vi "Read Heater and Valve.vi"(8 "error in (no error)":errorcluster, 11 "Temperature Controller in":refnum<class "Temperature Controller.lvclass">) -> (0 "error out":errorcluster, 1 "valve%":T2 caption="Valve" max=100.0 scale=0.0..100.0 scale format="%.1f", 2 "heater%":T2 caption="Heater" max=100.0 scale=0.0..100.0 scale format="%.1f", 3 "Temperature Controller out":refnum<class "Temperature Controller.lvclass">)   [LabVIEW 2012, in "Temperature Controller.lvclass"]
uses:
  Temperature Controller.lvclass
  HV Slide Indicator.ctl
  AutoCtl.ctl
  Temperature Controller.lvclass/Temperature Controller.ctl
panel:
  out "Auto":T1
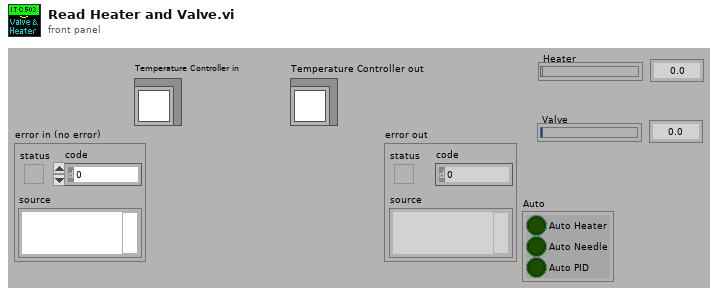
[diagram p1: front panel]
types:
  T1 = typedef "Temperature Controller.lvclass/AutoCtl.ctl" = cluster{"Auto Heater":bool, "Auto Needle":bool, "Auto PID":bool}
  T2 = typedef "Temperature Controller.lvclass/HV Slide Indicator.ctl" = dbl
  T3 = typedef "ITCIO.ctl" = cluster{"Address":T4, "Version":T5, "Ch 1 dec places":i16, "Ch 2 dec places":i16, "Ch 3 dec places":i16, "Ch1 Name":string, "Ch2 Name":string, "Ch3 Name":string}
  T4 = typedef "OxfordAddress.ctl" = cluster{"Com Port":i32, "ISOBUS Address":i32, "GPIB Address":i16, "Communication":enum16{"RS232", "ISOBUS", "GPIB", "Gateway"}}
  T5 = typedef "ITCVersion.ctl" = enum16{"ITC502", "ITC503", "ITC601"}
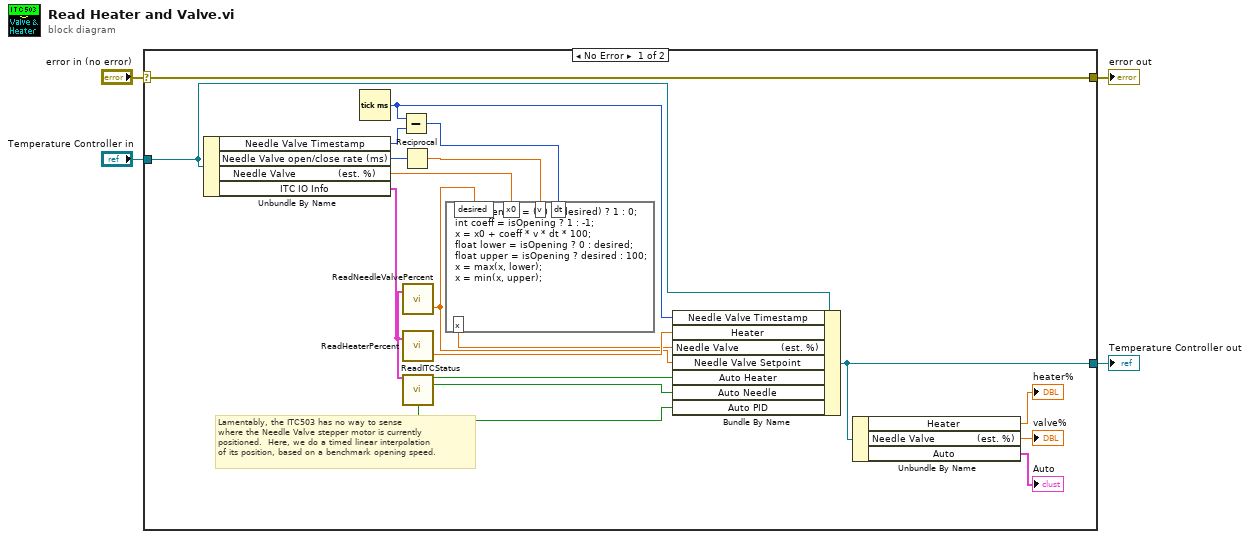
[diagram p0: block diagram]
diagram:
  n1 = case shown="No Error" "error in (no error)" {
    selector: "error in (no error)" -> [w6 w25]
    tunnel: "Temperature Controller in" -> [w16 w24]
    tunnel: [w10 w24] -> w3
    tunnel: [w6 w25] -> w2
    frame No Error {
      # "Lamentably, the ITC503 has no way to sense\nwhere the Needle Valve stepper motor is currently\npositioned.  Here, we do a timed linear interpolation\nof its position, based on a benchmark opening speed."
      n2 = Unbundle By Name(w16) -> ("Needle Valve Timestamp"=w15:u32, "Needle Valve open/close rate (ms)"=w14:u32, "Needle Valve              (est. %)"=w13:T2, "ITC IO Info"=w5:T3)
      n3 = Tick Count (ms)() -> (millisecond timer value=w12:u32)
      n4 = Subtract(x=w12, y=w15) -> (x-y=w22:u32)
      n5 = Reciprocal(x=w14) -> (1/x=w23:dbl)
      n6 = call "ReadNeedleValvePercent.vi"("IO Info"=w5) -> ("Actual Needle Valve  %"=w11:dbl)  [unwired: 2 out]
      n7 = call "ReadHeaterPercent.vi"("ITC IO Info"=w5) -> ("Actual heater  %"=w21:dbl)  [unwired: 2 out]
      n8 = call "ReadITCStatus.vi"("ITC IO Info"=w5) -> ("Auto heat"=w19:bool, "Auto Needle Valve"=w18:bool, "Auto PID"=w17:bool)  [unwired: 12 out]
      n9 = formula code="int isOpening = (x0 < desired) ? 1 : 0;\nint coeff = isOpening ? 1 : -1;\nx = x0 + coeff * v * dt * 100;\nfloat lower = isOpening ? 0 : desired;\nfloat upper = isOpening ? desired : 100;\nx = max(x, lower);\nx = min(x, upper);"("x0"=w13, "v"=w23, "dt"=w22, "desired"=w11) -> ("x"=w20:dbl)
      n10 = Bundle By Name(cluster=w16, "Needle Valve Timestamp"=w12, "Heater"=w21, "Needle Valve              (est. %)"=w20, "Needle Valve Setpoint"=w11, "Auto Heater"=w19, "Auto Needle"=w18, "Auto PID"=w17) -> (w10:refnum<class "Temperature Controller.lvclass">)
      n11 = Unbundle By Name(w10) -> ("Heater"=→"heater%":T2, "Needle Valve              (est. %)"=→"valve%":T2, "Auto"=→"Auto":T1)
    }
    frame Error {
    }
  }
  "Temperature Controller out" <- w3
  "error out" <- w2
